vi "Build Patrick Builder.vi"() -> ()   [LabVIEW 2019]
uses:
  <vilib>/Utility/sysdir.llb/System Directory Type.ctl
panel:
  out "string":string
  # "1. Configure build number and release notes with Patrick Builder.vipb\n\n2. Make desired changes to build.cfg or Inno.iss\n\n3. Run this VI\n\n4. Open a cmd window and paste and execute the following:"
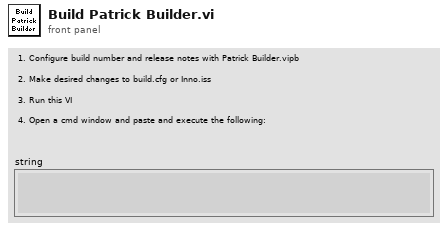
[diagram p1: front panel]
types:
  T1 = typedef "System Directory Type.ctl" = i32
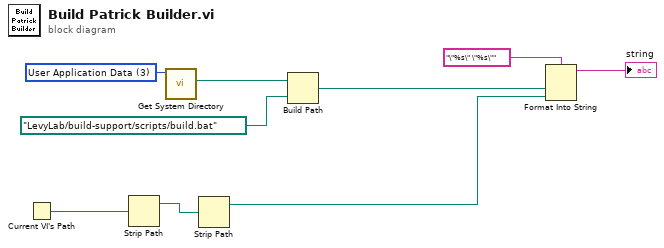
[diagram p0: block diagram]
diagram:
  w9 = T1 3 items=["User Home"=0, "User Desktop"=1, "User Documents"=2, "User Application Data"=3, "User Preferences"=4, "User Temporary"=5, "Public Documents"=6, "Public Application Data"=7, "Public Preferences"=8, "Public Cache"=13, "System Core Libraries"=9, "System Installed Libraries"=10, "Application Files"=11, "Boot Volume Root"=12] ("system directory type")
  n1 = Current VI's Path() -> (path=w3:path)
  n2 = Strip Path(path=w3) -> (stripped path=w2:path)  [unwired: 1 out]
  n3 = call <vilib>:"Get System Directory.vi"("system directory type"=w9) -> ("system directory"=w8:path)  [unwired: 10 in]
  n4 = Strip Path(path=w2) -> (stripped path=w1:path)  [unwired: 1 out]
  n5 = Build Path(base path=w8, name or relative path=path "LevyLab/build-support/scripts/build.bat") -> (appended path=w5:path)
  n6 = Format Into String(format string="\"%s\" \"%s\"", w5, w1) -> (resulting string=→"string":string)  [unwired: 2 in, 1 out]
